vi "CameraTriggerSetup.vi"(4 "Camera\nTrigger\nOutput":tag, 5 "Frame Rate":dbl, 6 "Sync Type":T2(ring), 7 "Exposure Time":dbl, 8 "error in":errorcluster, 9 "Camera\nClock\nCounter":tag, 10 "Start Trigger Source":tag, 11 "Exposure Start Delay":dbl) -> (0 "error out":errorcluster, 2 "CameraSignalDefinition":T1, 3 "CameraSignalRefnum":refnum<k21>)   [LabVIEW 2023]
uses:
  <vilib>/DAQmx/create/channels.llb/DAQmx Create Channel (CO-Pulse Generation-Time).vi
  <vilib>/DAQmx/configure/timing.llb/DAQmx Timing (Implicit).vi
  <vilib>/DAQmx/configure/trigger.llb/DAQmx Start Trigger (Digital Edge).vi
  <resource>/objmgr/daqmx.rc
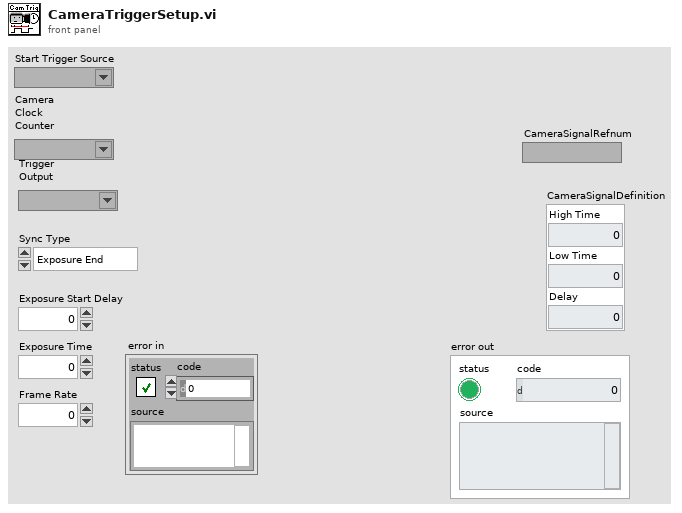
[diagram p1: front panel]
types:
  T1 = cluster{"High Time":dbl, "Low Time":dbl, "Delay":dbl}
  T2 = enum16{"Exposure End", "Exposure Center", "Exposure Start", "Start", "NoSync"}
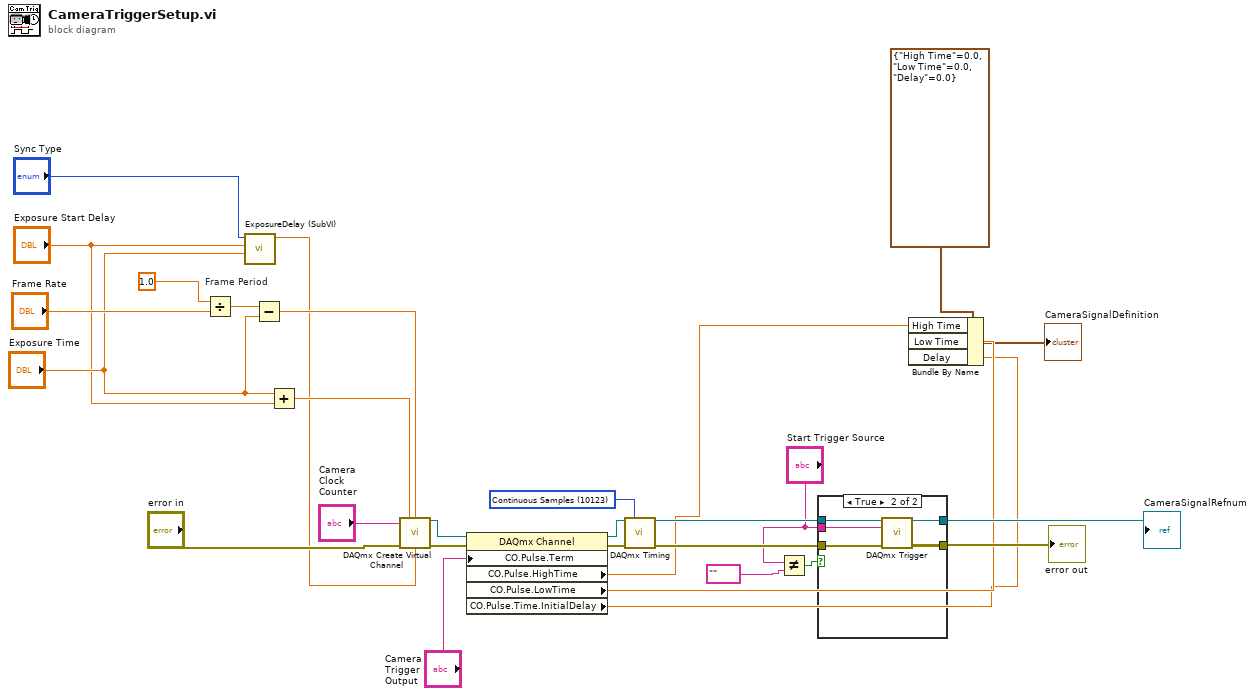
[diagram p0: block diagram]
diagram:
  w15 = 10123 items=["Finite Samples"=10178, "Continuous Samples"=10123, "Hardware Timed Single Point"=12522] ("sample mode")
  n1 = Divide "Frame Period"(x=1.0, y="Frame Rate") -> (x/y=w28:dbl)
  n2 = call "ExposureDelay (SubVI).vi"("Exposure Time"="Exposure Time", "Exposure Start Delay in"="Exposure Start Delay", "Enum"="Sync Type") -> ("Exposure Start Delay out"=w6:dbl)  [unwired: 8 in]
  n3 = Subtract(x=w28, y="Exposure Time") -> (x-y=w10:dbl)
  n4 = Add(x="Exposure Time", y="Exposure Start Delay") -> (x+y=w9:dbl)
  n5 = call-poly <vilib>:"DAQmx Create Virtual Channel.vi"("high time"=w9, "low time"=w10, "counter"="Camera\nClock\nCounter", "error in"="error in", "initial delay"=w6) -> ("task out"=w17:refnum<k21>, "error out"=w18:errorcluster)  [unwired: 9 in]
  n6 = property class="DAQmx Channel"(reference=w17, error in=w18, "CO.Pulse.Term"="Camera\nTrigger\nOutput") -> (reference out=w19:refnum<k21>, error out=w20:errorcluster, "CO.Pulse.HighTime"=w8:dbl, "CO.Pulse.LowTime"=w7:dbl, "CO.Pulse.Time.InitialDelay"=w5:dbl)
  n7 = call-poly <vilib>:"DAQmx Timing.vi"("task/channels in"=w19, "sample mode"=w15, "error in"=w20) -> ("task out"=w21:refnum<k21>, "error out"=w22:errorcluster)  [unwired: 11 in]
  n8 = Not Equal?(x="Start Trigger Source", y=tag "" ("Start Trigger Source 2")) -> (x != y?=w3:bool)
  n9 = case shown="True" w3 {
    tunnel: [w30 w36] -> w27
    tunnel: [w31 w35] -> w26
    tunnel: w22 -> [w30 w34]
    tunnel: w21 -> [w31 w33]
    tunnel: "Start Trigger Source" -> [_ w32]
    frame False {
    }
    frame True {
      n10 = call-poly <vilib>:"DAQmx Trigger.vi"("task/channels in"=w33, "source"=w32, "error in"=w34) -> ("task out"=w35:refnum<k21>, "error out"=w36:errorcluster)  [unwired: 11 in]
    }
  }
  "error out" <- w27
  "CameraSignalRefnum" <- w26
  n11 = Bundle By Name(cluster=T1 {"High Time"=0.0, "Low Time"=0.0, "Delay"=0.0}, "High Time"=w8, "Low Time"=w7, "Delay"=w5) -> (→"CameraSignalDefinition":T1)
